vi "initCanon.vi"() -> (0 "error out":errorcluster, 3 "inRef dup":u32)   [LabVIEW 2016]
uses:
  labview for canon om/Vital supporting file for labview program/LV-EDSDK-Distribution_0.2/Distribution/EDSDK-Labview.llb/kEdsProperties.ctl
  variables/applicationControl.vi
panel:
  out "outDeviceInfo":T1
  in  "error in (no error)":errorcluster
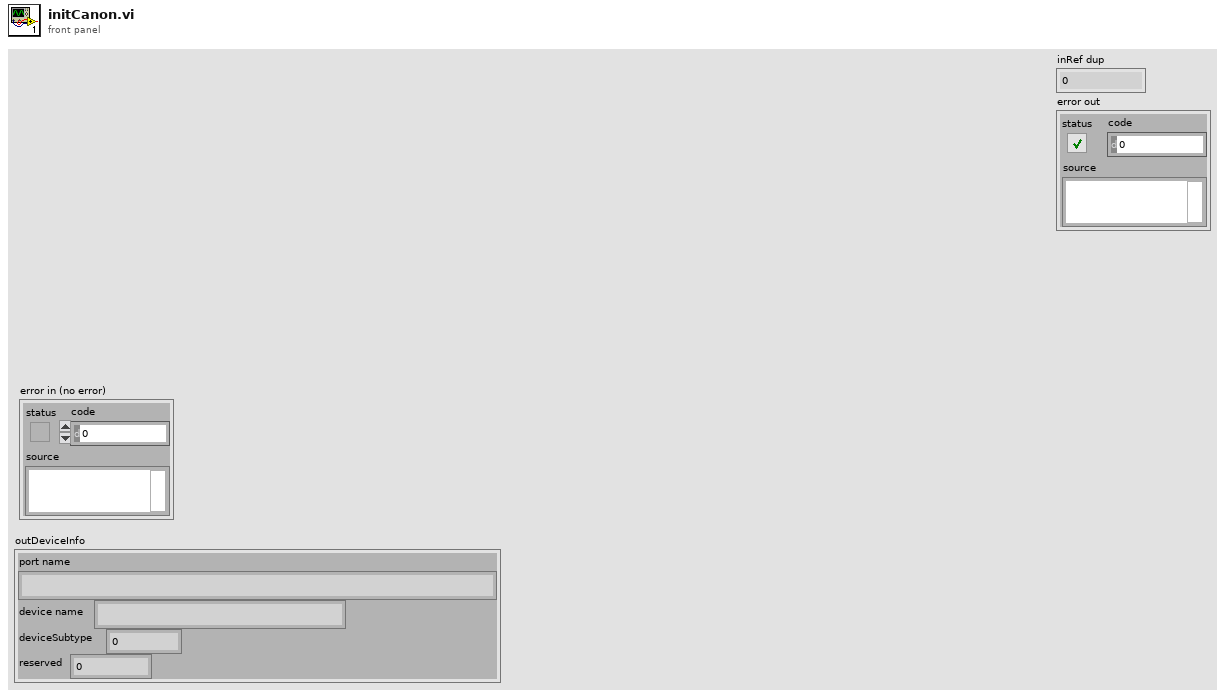
[diagram p1: front panel]
types:
  T1 = cluster{"port name":string, "device name":string, "deviceSubtype":u32, "reserved":u32}
  T2 = typedef "kEdsProperties.ctl" = u32
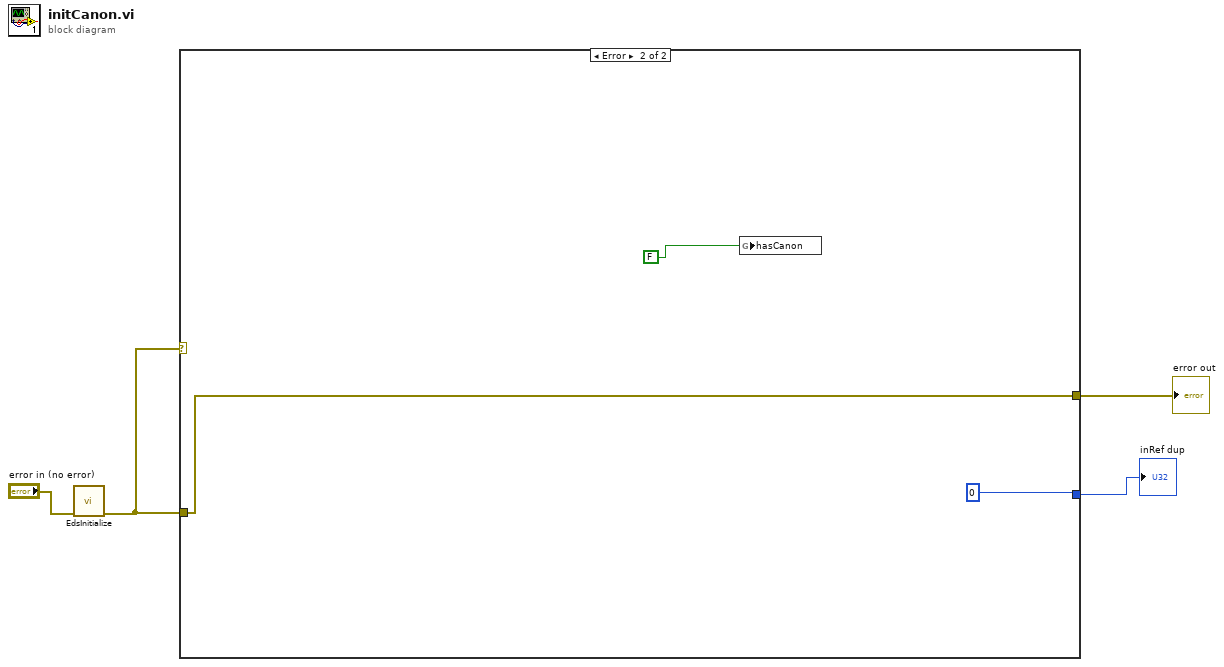
[diagram p0: block diagram]
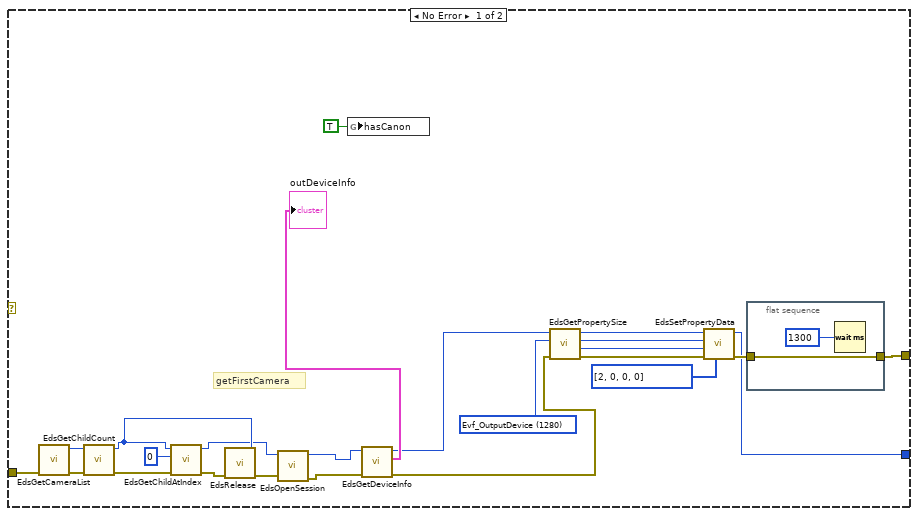
[diagram p2: hidden frame]
diagram:
  n1 = call "EdsInitialize.vi"("error in (no error)"="error in (no error)") -> ("error out"=w1:errorcluster)  [unwired: 10 in]
  n2 = case shown="Error" w1 {
    tunnel: w1 -> [w28 w33]
    tunnel: [w8 0] -> w3
    tunnel: [w6 w33] -> w2
    frame No Error {
      w10 = T2 1280 items=["Unknown"=65535, "ProductName"=2, "BodyID"=3, "OwnerName"=4, "MakerName"=5, "DateTime"=6, "FirmwareVersion"=7, "BatteryLevel"=8, "CFn"=9, "SaveTo"=11, "CurrentStorage"=12, "CurrentFolder"=13, "MyMenu"=14, "BatteryQuality"=16, "HDDirectoryStructure"=32, "ImageQuality"=256, "JpegQuality"=257, "Orientation"=258, "ICCProfile"=259, "FocusInfo"=260, "DigitalExposure"=261, "WhiteBalance"=262, "ColorTemperature"=263, "WhiteBalanceShift"=264, "Contrast"=265, "ColorSaturation"=266, "ColorTone"=267, "Sharpness"=268, "ColorSpace"=269, "ToneCurve"=270, "PhotoEffect"=271, "FilterEffect"=272, "ToningEffect"=273, "ParameterSet"=274, "ColorMatrix"=275, "PictureStyle"=276, "PictureStyleDesc"=277, "ETTL2Mode"=279, "PictureStyleCaption"=512, "Linear"=768, "ClickWBPoint"=769, "WBCoeffs"=770, "GPSVersionID"=2048, "GPSLatitudeRef"=2049, "GPSLatitude"=2050, "GPSLongitudeRef"=2051, "GPSLongitude"=2052, "GPSAltitudeRef"=2053, "GPSAltitude"=2054, "GPSTimeStamp"=2055, "GPSSatellites"=2056, "GPSStatus"=2057, "GPSMapDatum"=2066, "GPSDateStamp"=2077, "AtCapture_Flag"=2147483648, "AEMode"=1024, "DriveMode"=1025, "ISOSpeed"=1026, "MeteringMode"=1027, "AFMode"=1028, "Av"=1029, "Tv"=1030, "ExposureCompensation"=1031, "FlashCompensation"=1032, "FocalLength"=1033, "AvailableShots"=1034, "Bracket"=1035, "WhiteBalanceBracket"=1036, "LensName"=1037, "AEBracket"=1038, "FEBracket"=1039, "ISOBracket"=1040, "NoiseReduction"=1041, "FlashOn"=1042, "RedEye"=1043, "FlashMode"=1044, "LensStatus"=1046, "Artist"=1048, "Copyright"=1049, "DepthOfField"=1051, "EFCompensation"=1054, "Evf_OutputDevice"=1280, "Evf_Mode"=1281, "Evf_WhiteBalance"=1282, "Evf_ColorTemperature"=1283, "Evf_DepthOfFieldPreview"=1284, "Evf_Zoom"=1287, "Evf_ZoomPosition"=1288, "Evf_FocusAid"=1289, "Evf_Histogram"=1290, "Evf_ImagePosition"=1291, "Evf_HistogramStatus"=1292, "Evf_AFMode"=1294, "Evf_CoordinateSystem"=1344, "Evf_ZoomRect"=1345] ("inPropertyID")
      # "getFirstCamera"
      n3 = call "EdsGetCameraList.vi"("error in"=w28) -> ("error out"=w27:errorcluster, "outCameraListRef"=w23:u32)  [unwired: 9 in]
      n4 = call "EdsGetChildCount.vi"("error in"=w27, "inRef"=w23) -> ("error out"=w26:errorcluster, "inRef dup"=w22:u32)  [unwired: 7 in, 1 out]
      n5 = call "EdsGetChildAtIndex.vi"("error in"=w26, "index"=u32 0, "inRef"=w22) -> ("error out"=w24:errorcluster, "outRef"=w18:u32)  [unwired: 7 in]
      n6 = call "EdsRelease.vi"("error in"=w24, "inRef"=w22) -> ("error out"=w21:errorcluster)  [unwired: 7 in, 2 out]
      n7 = call "EdsOpenSession.vi"("error in"=w21, "inCameraRef"=w18) -> ("error out"=w19:errorcluster, "inCameraRef dup"=w20:u32)  [unwired: 8 in]
      n8 = global write "applicationControl.vi" "hasCanon"(TRUE ("hasCanon")) -> ()
      n9 = call "EdsGetDeviceInfo.vi"("error in"=w19, "inCameraRef"=w20) -> ("error out"=w7:errorcluster, "outDeviceInfo"=→"outDeviceInfo":T1, "inCameraRef dup"=w9:u32)  [unwired: 7 in]
      n10 = call "EdsGetPropertySize.vi"("error in"=w7, "inPropertyID"=w10, "inRef"=w9) -> ("error out"=w13:errorcluster, "outSize"=w14:u32, "inPropertyID dup"=w12:T2, "inRef dup"=w11:u32)  [unwired: 4 in, 1 out]
      n11 = call "EdsSetPropertyData.vi"("inPropertyData"=u8[] [2, 0, 0, 0], "error in"=w13, "inPropertySize"=w14, "inPropertyID"=w12, "inRef"=w11) -> ("error out"=w16:errorcluster, "inRef dup"=w8:u32)  [unwired: 5 in]
      n12 = flat-sequence {
        tunnel: w16 -> [w30]
        tunnel: [w30] -> w6
        frame #0 {
          n13 = Wait (ms)(milliseconds to wait=u32 1300) -> ()  [unwired: 1 out]
        }
      }
    }
    frame Error {
      n14 = global write "applicationControl.vi" "hasCanon"(FALSE) -> ()
    }
  }
  "inRef dup" <- w3
  "error out" <- w2
